vi "U16ToType.vi"(4 "U16 In":u16) -> (1 "Type out":T1=enum."RATIONAL")   [LabVIEW 2015, in "Tiff reader.lvlib"]
doc: "Converts U8 to data type."
uses:
  Tiff reader.lvlib
  FieldTypes.ctl
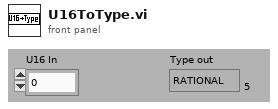
[diagram p1: front panel]
types:
  T1 = typedef "Tiff reader.lvlib/FieldTypes.ctl" = enum16{"NULL", "U8", "ASCII7", "U16", "U32", "RATIONAL", "SByte(I8)", "Undef(8Bit)", "I16", "I32", "SRat(4B:4B)", "SGL(4Byte)", "DBL(8Byte)"}
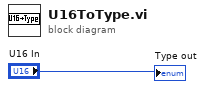
[diagram p0: block diagram]
diagram:
  "Type out" <- "U16 In"
